vi "Marker Mode.vi"(5 "Marker (1)":i32=1, 6 "Marker Mode (T: Discrete)":bool=TRUE, 7 "Channel (1)":i32=1, 8 "error in (no error)":errorcluster, 9 "Reference Marker Mode (F: Disable)":bool, 10 "Coupled (F: Disable)":bool, 11 "VISA resource name":refnum<visa-resource-name>) -> (0 "error out":errorcluster, 3 "VISA resource name out":refnum<visa-resource-name>)   [LabVIEW 2011, in "Agilent ENA Series.lvlib"]
doc: "This VI configures marker mode."
uses:
  Agilent ENA Series.lvlib
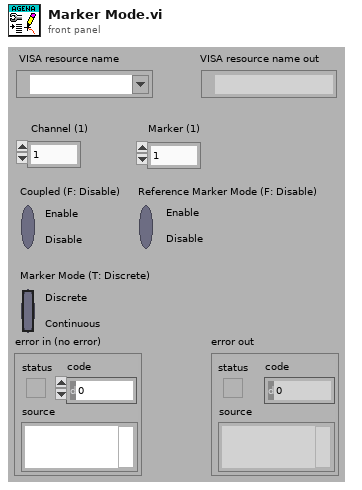
[diagram p1: front panel]
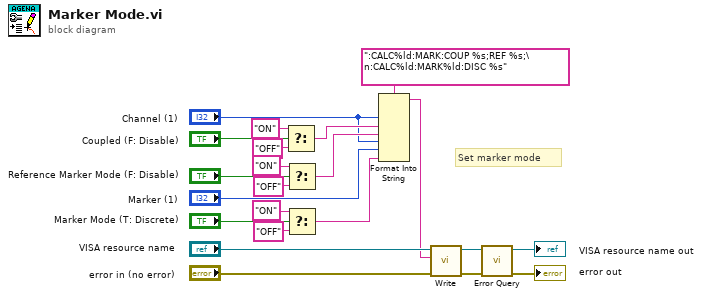
[diagram p0: block diagram]
diagram:
  # "Set marker mode"
  n1 = Select(t="ON", s="Coupled (F: Disable)", f="OFF") -> (s? t:f=w15:string)
  n2 = Select(t="ON", s="Reference Marker Mode (F: Disable)", f="OFF") -> (s? t:f=w8:string)
  n3 = Select(t="ON", s="Marker Mode (T: Discrete)", f="OFF") -> (s? t:f=w5:string)
  n4 = Format Into String(format string=":CALC%ld:MARK:COUP %s;REF %s;\n:CALC%ld:MARK%ld:DISC %s", "Channel (1)", w15, w8, "Channel (1)", "Marker (1)", w5) -> (resulting string=w19:string)  [unwired: 2 in, 1 out]
  n5 = call "Write.vi"("error in (no error)"="error in (no error)", "String ()"=w19, "VISA resource name"="VISA resource name") -> ("error out"=w3:errorcluster, "VISA resource name out"=w4:refnum<visa-resource-name>)  [unwired: 6 in, 1 out]
  n6 = call "Error Query.vi"("error in (no error)"=w3, "VISA resource name"=w4) -> ("error out"=→"error out":errorcluster, "VISA resource name out"=→"VISA resource name out":refnum<visa-resource-name>)  [unwired: 6 in, 2 out]
